vi "Call_Edge.vi"(0 "Mode":bool, 5 "Call_Edge":bool, 11 "Error_In":errorcluster) -> (15 "Error_Out":errorcluster)   [LabVIEW 2021]
doc: "This VI can be used to launch Soliton technologies website in edge."
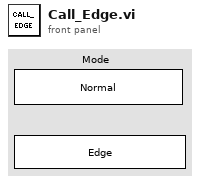
[diagram p1: front panel]
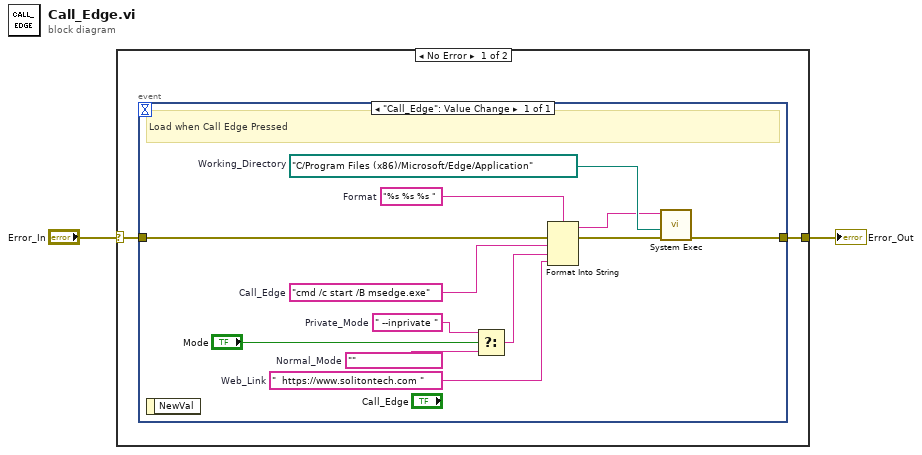
[diagram p0: block diagram]
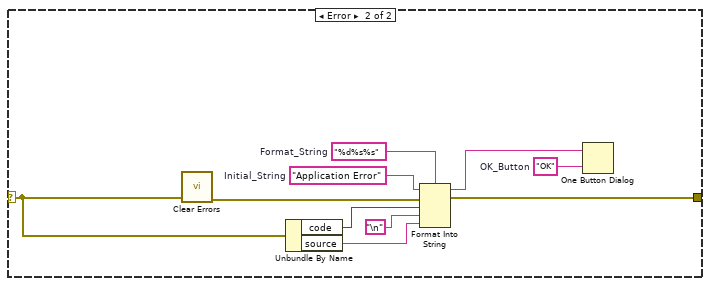
[diagram p2: hidden frame]
diagram:
  n1 = case shown="No Error" "Error_In" {
    selector: "Error_In" -> [w4 w20]
    tunnel: [w3 w19] -> w1
    frame No Error {
      n2 = event shown="[0] \"Call_Edge\": Value Change" {
        selector: _ -> [_]
        dyn-events: _ -> [_]
        timeout: _ -> [_]
        tunnel: w4 -> [w15]
        tunnel: [w14] -> w3
        event "Call_Edge": Value Change {
          w8 = ""  # Normal_Mode
          w7 = "  https://www.solitontech.com "  # Web_Link
          w9 = " --inprivate "  # Private_Mode
          w11 = "cmd /c start /B msedge.exe"  # Call_Edge
          w12 = "%s %s %s "  # Format
          w16 = path "C:/Program Files (x86)/Microsoft/Edge/Application"  # Working_Directory
          # "Load when Call Edge Pressed"
          n3 = event-data() -> ()  [unwired: 1 in, 1 out]
          n4 = Select(t=w9, s="Mode", f=w8) -> (s? t:f=w10:string)
          n5 = Format Into String(format string=w12, error in=w15, w11, w10, w7) -> (resulting string=w6:string, error out=w13:errorcluster)  [unwired: 1 in]
          n6 = call <vilib>:"System Exec.vi"("error in (no error)"=w13, "working directory"=w16, "command line"=w6) -> ("error out"=w14:errorcluster)  [unwired: 5 in, 3 out]
        }
      }
    }
    frame Error {
      w25 = "%d%s%s"  # Format_String
      w26 = "Application Error"  # Initial_String
      w17 = "OK"  # OK_Button
      n7 = call <vilib>:"Clear Errors.vi"("error in (no error)"=w20) -> ("error out"=w23:errorcluster)  [unwired: 5 in, 1 out]
      n8 = Unbundle By Name(w20) -> ("code"=w22:i32, "source"=w21:string)
      n9 = Format Into String(format string=w25, initial string=w26, error in=w23, w22, "\n", w21) -> (resulting string=w18:string, error out=w19:errorcluster)
      n10 = One Button Dialog(message=w18, button name ("OK")=w17) -> ()  [unwired: 1 out]
    }
  }
  "Error_Out" <- w1
